vi "Msg.vi"(7 "Actor in":refnum<class "Actor.lvclass">, 11 "Set Error Msg in":refnum<class "Set Error Msg.lvclass">) -> (5 "Actor out":refnum<class "Actor.lvclass">)   [LabVIEW 2021, in "Set Error.lvlib" / "Set Error Msg.lvclass"]
uses:
  Set Error Msg.lvclass
  jettl/Actor/Actor.lvclass
  Set Error/Set Error.lvclass
  768161d2-33f0-48d3-a999-7da2b215e45b.vi
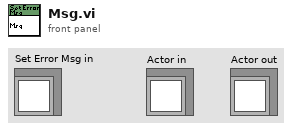
[diagram p1: front panel]
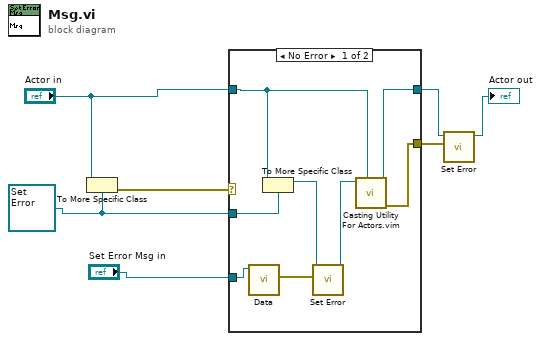
[diagram p0: block diagram]
diagram:
  w1 = refnum<class "Set Error.lvclass"> refnum ("Error.lvlib:Error.lvclass")
  n1 = To More Specific Class(target class=w1, reference="Actor in") -> (error out=w7:errorcluster)  [unwired: 1 in, 1 out]
  n2 = case shown="No Error" w7 {
    selector: w7 -> [_ w16]
    tunnel: [w14 w17] -> w6
    tunnel: "Actor in" -> [w13 w17]
    tunnel: w1 -> [w15 _]
    tunnel: "Set Error Msg in" -> [w11 _]
    tunnel: [w12 w16] -> w5
    frame No Error {
      n3 = call "Data.vi"("Set Error Msg in"=w11) -> ("Error"=w10:errorcluster)  [unwired: 10 in]
      n4 = To More Specific Class(target class=w15, reference=w13) -> (specific class reference=w9:refnum<class "Set Error.lvclass">)  [unwired: 1 in, 1 out]
      n5 = call-dynamic "Set Error.vi"("Error"=w10, "Set Error in"=w9) -> ("Set Error out"=w8:refnum<class "Set Error.lvclass">)  [unwired: 9 in]
      n6 = call "Casting Utility For Actors.vim"("type"=w13, "Actor in"=w8) -> ("error out"=w12:errorcluster, "Actor out"=w14:refnum<class "Actor.lvclass">)  [unwired: 8 in]
    }
    frame Error {
    }
  }
  n7 = call-dynamic "Set Error.vi"("Error"=w5, "Actor in"=w6) -> ("Actor out"=→"Actor out":refnum<class "Actor.lvclass">)  [unwired: 9 in]
